vi "Constants.vi"() -> ()   [LabVIEW 2017, in "TreeSerializer.lvlib"]
uses:
  TreeSerializer.lvlib
panel:
  in  "DisabledName":string="Disabled"
  in  "ChildrenName":string="Children"
  in  "PathName":string="Path"
  in  "VIName":string="VIName"
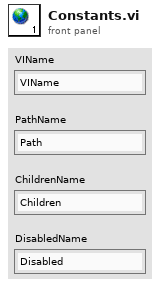
[diagram p1: front panel]
diagram:
